vi "Tango Reset.vi"(8 "error in (no error)":errorcluster, 10 "XYZ notifier":refnum<notifier>, 11 "Queue in":refnum<queue>) -> (0 "error out":errorcluster, 2 "Measurements":dbl[](array[numeric]), 3 "Position":cluster{"dX":dbl, "dY":dbl, "dZ":dbl, "dA":dbl})   [LabVIEW 2020]
uses:
  Message Queue/Message Cluster.ctl
  Message Queue/Message Queue.lvlib
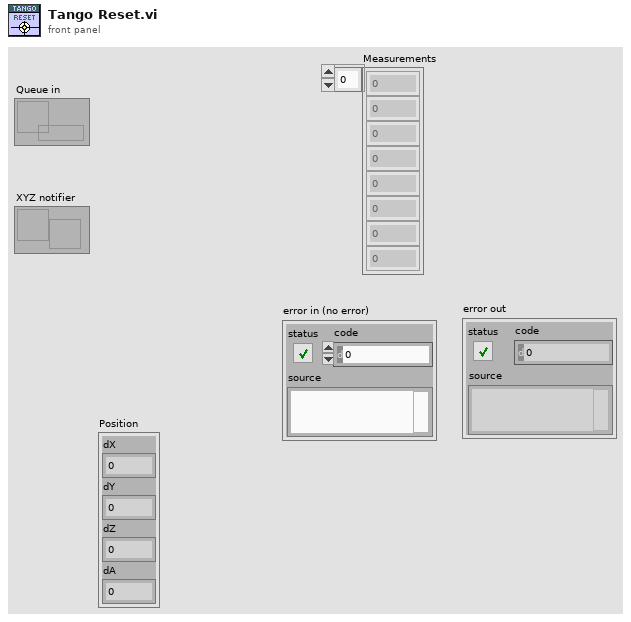
[diagram p1: front panel]
types:
  T1 = cluster{"Next Step":string, "Trigger Level":dbl, "Timebase":dbl, "Source (0: Channel 1) 2":u16[]}
  T2 = cluster{"Type CMD":string, "Mode CMD":string, "Main CMD":string}
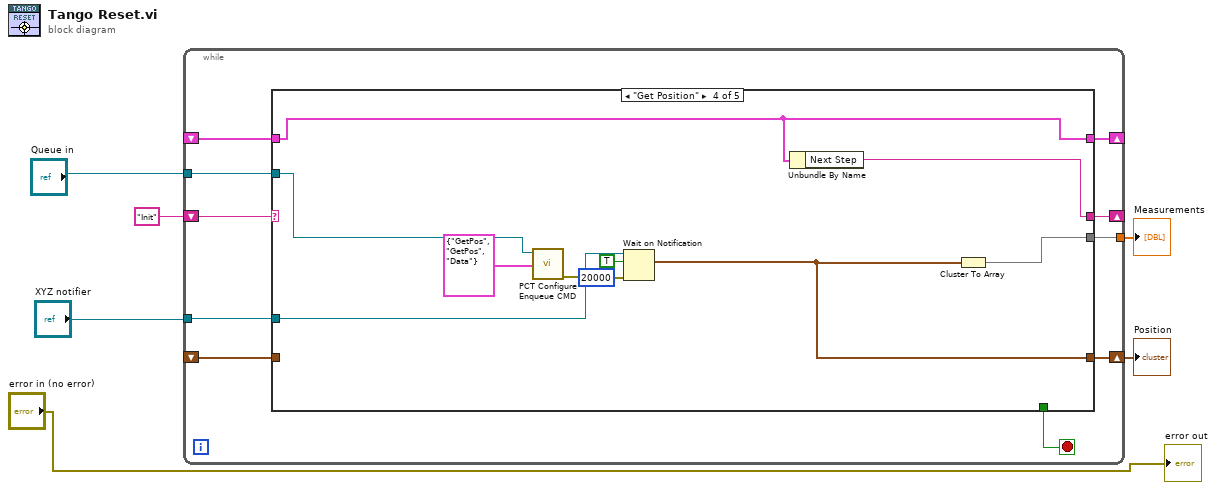
[diagram p0: block diagram]
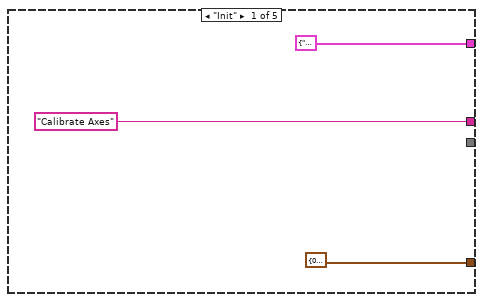
[diagram p2: hidden frame]
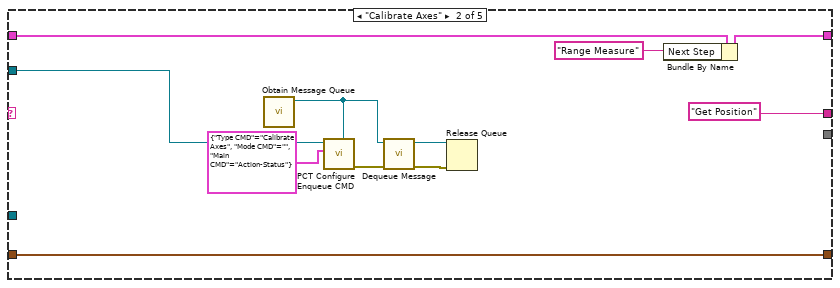
[diagram p3: hidden frame]
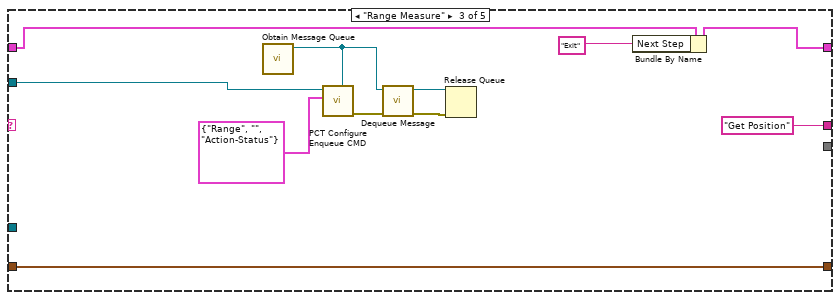
[diagram p4: hidden frame]
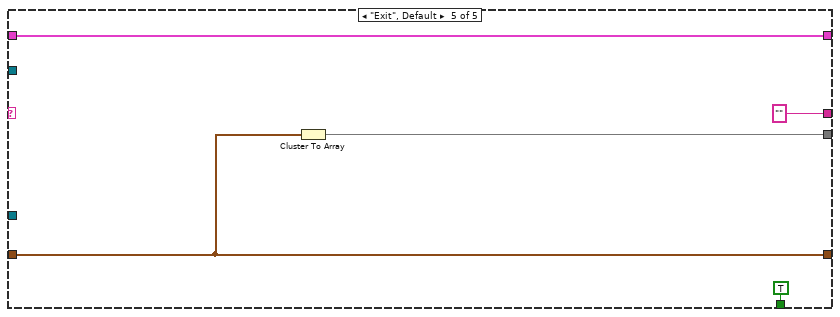
[diagram p5: hidden frame]
diagram:
  n1 = while {
    shift-right: [w15] -> _
    shift-left: "Init" -> [w16]
    shift-right: [w14] -> _
    shift-left: _ -> [w13]
    tunnel: "Queue in" -> [w12]
    tunnel: "XYZ notifier" -> [w10]
    shift-right: [w9] -> w3
    shift-left: _ -> [w8]
    tunnel: [w7] -> w2
    stop <- w11 stop-if-true
    n2 = case shown="\"Get Position\"" w16 {
      tunnel: ["Calibrate Axes" "Get Position" "Get Position" ("Next Step") w42 "" ("Next Step")] -> w15
      tunnel: [T1 {"Next Step"="Configure Scope", "Trigger Level"=2.0, "Timebase"=0.1, "Source (0: Channel 1) 2"=[0, 1, 2]} w21 w32 w43 w54] -> w14
      tunnel: w13 -> [_ w30 w41 w43 w54]
      tunnel: w12 -> [_ w27 w33 w50 _]
      tunnel: [_ _ _ _ TRUE] -> w11
      tunnel: w10 -> [_ _ _ w48 _]
      tunnel: [cluster{"dX":dbl, "dY":dbl, "dZ":dbl, "dA":dbl} {"dX"=0.0, "dY"=0.0, "dZ"=0.0, "dA"=0.0} ("notification") w28 w40 w46 w53] -> w9
      tunnel: w8 -> [_ w28 w40 _ w53]
      tunnel: [_ _ _ w49 w52] -> w7
      frame "Init" {
      }
      frame "Calibrate Axes" {
        n3 = call "Obtain Message Queue.vi"() -> ("Message Queue"=w24:refnum<queue>)  [unwired: 10 in, 1 out]
        n4 = call "PCT Configure Enqueue CMD.vi"("Response Queue"=w24, "CMD"=T2 {"Type CMD"="Calibrate Axes", "Mode CMD"="", "Main CMD"="Action-Status"}, "CMD Queue in"=w27) -> ("error out"=w25:errorcluster)  [unwired: 6 in, 2 out]
        n5 = call "Dequeue Message.vi"("error in (no error)"=w25, "Message Queue"=w24) -> ("error out"=w23:errorcluster, "dup Message Queue"=w22:refnum<queue>)  [unwired: 6 in, 2 out]
        n6 = Release Queue(queue=w22, error in (no error)=w23) -> ()  [unwired: 1 in, 3 out]
        n7 = Bundle By Name(cluster=w30, "Next Step"="Range Measure") -> (w21:T1)
      }
      frame "Range Measure" {
        n8 = call "Obtain Message Queue.vi"() -> ("Message Queue"=w37:refnum<queue>)  [unwired: 10 in, 1 out]
        n9 = call "PCT Configure Enqueue CMD.vi"("Response Queue"=w37, "CMD"=T2 {"Type CMD"="Range", "Mode CMD"="", "Main CMD"="Action-Status"}, "CMD Queue in"=w33) -> ("error out"=w38:errorcluster)  [unwired: 6 in, 2 out]
        n10 = call "Dequeue Message.vi"("error in (no error)"=w38, "Message Queue"=w37) -> ("error out"=w36:errorcluster, "dup Message Queue"=w35:refnum<queue>)  [unwired: 6 in, 2 out]
        n11 = Release Queue(queue=w35, error in (no error)=w36) -> ()  [unwired: 1 in, 3 out]
        n12 = Bundle By Name(cluster=w41, "Next Step"="Exit") -> (w32:T1)
      }
      frame "Get Position" {
        n13 = call "PCT Configure Enqueue CMD.vi"("CMD"=T2 {"Type CMD"="GetPos", "Mode CMD"="GetPos", "Main CMD"="Data"}, "CMD Queue in"=w50) -> ("error out"=w47:errorcluster)  [unwired: 7 in, 2 out]
        n14 = Wait on Notification(notifier=w48, ignore previous (F)=TRUE, timeout in ms (-1)=20000, error in (no error)=w47) -> (notification=w46:cluster{"dX":dbl, "dY":dbl, "dZ":dbl, "dA":dbl})  [unwired: 3 out]
        n15 = Unbundle By Name(w43) -> ("Next Step"=w42:string)
        n16 = Cluster To Array(cluster=w46) -> (array=w49:dbl[])
      }
      frame "Exit", Default {
        n17 = Cluster To Array(cluster=w53) -> (array=w52:dbl[])
      }
    }
  }
  "Position" <- w3
  "Measurements" <- w2
  "error out" <- "error in (no error)"
